vi "Load Bootstrap Config.vi"(8 "error in":errorcluster, 11 "Framework Engine in":refnum<class "Framework Engine.lvclass">) -> (0 "error out":errorcluster, 3 "Framework Engine out":refnum<class "Framework Engine.lvclass">)   [LabVIEW 2026, in "Framework Engine.lvclass"]
uses:
  Framework Engine.lvclass
  Framework Engine.lvclass/Framework Engine.ctl
  Services/Settings Service/Settings Service.lvclass
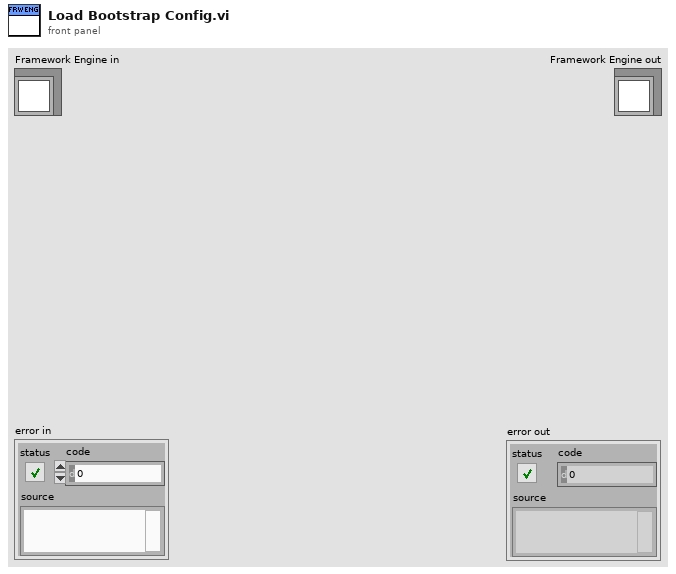
[diagram p1: front panel]
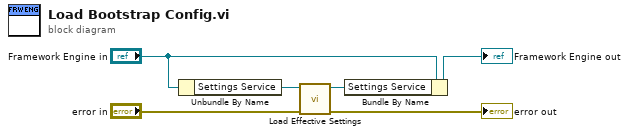
[diagram p0: block diagram]
diagram:
  n1 = Unbundle By Name("Framework Engine in") -> ("Settings Service"=w6:refnum<class "Settings Service.lvclass">)
  n2 = call "Load Effective Settings.vi"("error in"="error in", "Settings Service in"=w6) -> ("error out"=→"error out":errorcluster, "Setting Service out"=w3:refnum<class "Settings Service.lvclass">)  [unwired: 8 in]
  n3 = Bundle By Name(cluster="Framework Engine in", "Settings Service"=w3) -> (→"Framework Engine out":refnum<class "Framework Engine.lvclass">)
